vi "Line by Line Parsing Examples.vi"() -> ()   [LabVIEW 2022 SP3]
uses:
  <vilib>/regexp/Match Regular Expression.xnode
panel:
  out "Array":T1(array[cluster])
  out "before substring":string
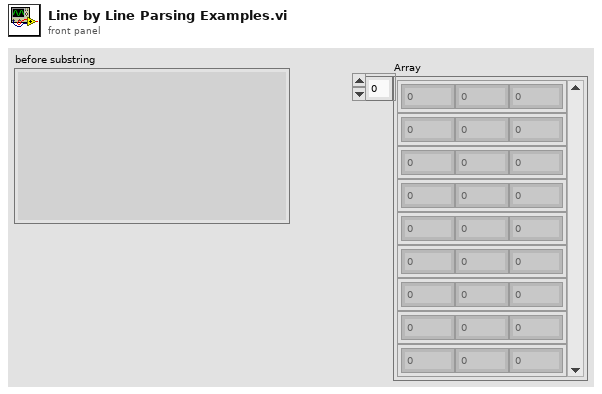
[diagram p1: front panel]
types:
  T1 = cluster{"submatch 1":i32, "submatch 2":i32, "submatch 3":i32}[]
  T2 = cluster{"submatch 1":string, "submatch 2":string, "submatch 3":string}
  T3 = cluster{"submatch 1":i32, "submatch 2":i32, "submatch 3":i32}
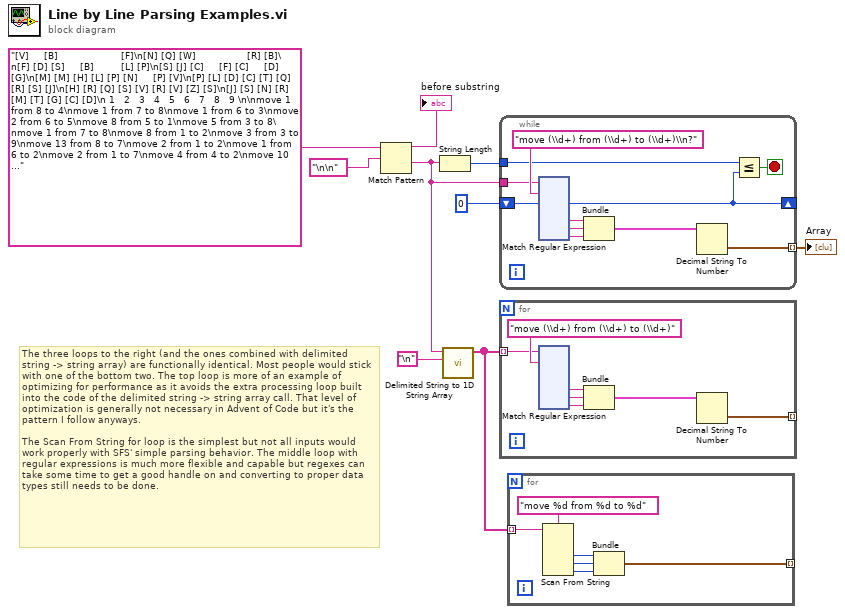
[diagram p0: block diagram]
diagram:
  # "The three loops to the right (and the ones combined with delimited string -> string array) are functionally identical. Most people would stick with one of the bottom two. The top loop is more of an example of optimizing for performance as it avoids the extra processing loop built into the code of the delimited string -> string array call. That level of optimization is generally not necessary in Advent of Code but it's the pattern I follow anyways.\n\nThe Scan From String for loop is the simplest but not all inputs would work properly with SFS' simple parsing behavior. The middle loop with regular expressions is much more flexible and capable but regexes can take some time to get a good handle on and converting to proper data types still needs to be done."
  n1 = Match Pattern(string="[V]     [B]                     [F]\n[N] [Q] [W]                 [R] [B]\n[F] [D] [S]     [B]         [L] [P]\n[S] [J] [C]     [F] [C]     [D] [G]\n[M] [M] [H] [L] [P] [N]     [P] [V]\n[P] [L] [D] [C] [T] [Q] [R] [S] [J]\n[H] [R] [Q] [S] [V] [R] [V] [Z] [S]\n[J] [S] [N] [R] [M] [T] [G] [C] [D]\n 1   2   3   4   5   6   7   8   9 \n\nmove 1 from 8 to 4\nmove 1 from 7 to 8\nmove 1 from 6 to 3\nmove 2 from 6 to 5\nmove 8 from 5 to 1\nmove 5 from 3 to 8\nmove 1 from 7 to 8\nmove 8 from 1 to 2\nmove 3 from 3 to 9\nmove 13 from 8 to 7\nmove 2 from 1 to 2\nmove 1 from 6 to 2\nmove 2 from 1 to 7\nmove 4 from 4 to 2\nmove 10 from 9 to 4\nmove 7 from 4 to 1\nmove 1 from 6 to 7\nmove 2 from 4 to 5\nmove 1 from 5 to 2\nmove 1 from 5 to 8\nmove 3 from 1 to 5\nmove 2 from 4 to 6\nmove 2 from 6 to 4\nmove 2 from 4 to 5\nmove 5 from 1 to 5\nmove 1 from 9 to 5\nmove 1 from 8 to 5\nmove 14 from 2 to 6\nmove 12 from 7 to 4\nmove 4 from 6 to 7\nmove 3 from 6 to 4\nmove 4 from 4 to 9\nmove 2 from 4 to 6\nmove 2 from 9 to 3\nmove 9 from 4 to 3\nmove 2 from 1 to 6\nmove 5 from 7 to 3\nmove 4 from 7 to 8\nmove 2 from 6 to 7\nmove 3 from 6 to 7\nmove 10 from 5 to 8\nmove 8 from 8 to 9\nmove 10 from 9 to 7\nmove 12 from 7 to 5\nmove 1 from 1 to 5\nmove 3 from 7 to 2\nmove 10 from 3 to 7\nmove 6 from 5 to 7\nmove 2 from 6 to 1\nmove 12 from 2 to 7\nmove 3 from 3 to 1\nmove 1 from 6 to 5\nmove 10 from 5 to 7\nmove 3 from 3 to 4\nmove 34 from 7 to 1\nmove 2 from 6 to 9\nmove 1 from 6 to 3\nmove 3 from 1 to 3\nmove 1 from 7 to 3\nmove 3 from 3 to 6\nmove 1 from 4 to 3\nmove 22 from 1 to 6\nmove 2 from 9 to 7\nmove 2 from 4 to 9\nmove 12 from 6 to 8\nmove 1 from 7 to 6\nmove 4 from 8 to 2\nmove 1 from 7 to 1\nmove 6 from 8 to 9\nmove 1 from 2 to 5\nmove 1 from 2 to 7\nmove 13 from 1 to 2\nmove 2 from 3 to 1\nmove 4 from 7 to 5\nmove 3 from 9 to 4\nmove 1 from 1 to 8\nmove 4 from 5 to 2\nmove 12 from 6 to 2\nmove 3 from 1 to 3\nmove 1 from 4 to 1\nmove 9 from 8 to 5\nmove 6 from 5 to 7\nmove 2 from 4 to 5\nmove 5 from 9 to 6\nmove 5 from 3 to 7\nmove 30 from 2 to 6\nmove 11 from 7 to 9\nmove 36 from 6 to 3\nmove 10 from 9 to 3\nmove 1 from 6 to 5\nmove 3 from 5 to 2\nmove 2 from 5 to 2\nmove 28 from 3 to 4\nmove 6 from 4 to 1\nmove 1 from 2 to 3\nmove 2 from 5 to 2\nmove 6 from 1 to 7\nmove 1 from 1 to 6\nmove 6 from 3 to 5\nmove 6 from 7 to 2\nmove 1 from 6 to 4\nmove 2 from 2 to 6\nmove 8 from 2 to 1\nmove 3 from 2 to 4\nmove 2 from 3 to 4\nmove 4 from 3 to 4\nmove 1 from 6 to 1\nmove 2 from 1 to 8\nmove 1 from 6 to 4\nmove 1 from 9 to 3\nmove 2 from 5 to 4\nmove 1 from 8 to 7\nmove 1 from 7 to 9\nmove 1 from 3 to 5\nmove 1 from 8 to 6\nmove 34 from 4 to 9\nmove 13 from 9 to 8\nmove 1 from 8 to 2\nmove 1 from 2 to 1\nmove 4 from 5 to 1\nmove 9 from 8 to 7\nmove 11 from 1 to 3\nmove 1 from 4 to 2\nmove 1 from 6 to 7\nmove 1 from 9 to 4\nmove 1 from 4 to 1\nmove 1 from 5 to 3\nmove 5 from 7 to 8\nmove 1 from 2 to 5\nmove 1 from 5 to 1\nmove 21 from 9 to 5\nmove 19 from 3 to 4\nmove 17 from 4 to 6\nmove 2 from 8 to 4\nmove 2 from 6 to 8\nmove 2 from 6 to 9\nmove 2 from 7 to 6\nmove 1 from 4 to 9\nmove 6 from 5 to 6\nmove 1 from 9 to 8\nmove 8 from 5 to 7\nmove 15 from 6 to 2\nmove 1 from 9 to 7\nmove 2 from 1 to 6\nmove 3 from 4 to 7\nmove 1 from 1 to 6\nmove 3 from 5 to 4\nmove 2 from 5 to 6\nmove 2 from 4 to 1\nmove 13 from 7 to 8\nmove 2 from 6 to 4\nmove 3 from 2 to 4\nmove 2 from 7 to 6\nmove 5 from 4 to 6\nmove 4 from 2 to 6\nmove 1 from 1 to 9\nmove 18 from 8 to 3\nmove 1 from 4 to 5\nmove 1 from 2 to 7\nmove 15 from 3 to 1\nmove 1 from 5 to 1\nmove 3 from 3 to 4\nmove 1 from 5 to 4\nmove 1 from 5 to 6\nmove 1 from 6 to 8\nmove 2 from 8 to 2\nmove 3 from 1 to 8\nmove 6 from 2 to 8\nmove 1 from 7 to 6\nmove 12 from 8 to 5\nmove 2 from 9 to 6\nmove 6 from 1 to 5\nmove 9 from 5 to 3\nmove 1 from 2 to 8\nmove 20 from 6 to 9\nmove 3 from 6 to 7\nmove 1 from 7 to 1\nmove 7 from 3 to 4\nmove 2 from 7 to 2\nmove 1 from 8 to 7\nmove 8 from 4 to 1\nmove 11 from 1 to 7\nmove 10 from 7 to 6\nmove 2 from 4 to 9\nmove 21 from 9 to 3\nmove 6 from 5 to 9\nmove 6 from 3 to 2\nmove 1 from 4 to 5\nmove 1 from 7 to 9\nmove 8 from 3 to 2\nmove 9 from 2 to 1\nmove 14 from 1 to 6\nmove 1 from 1 to 7\nmove 4 from 3 to 8\nmove 3 from 8 to 7\nmove 5 from 7 to 4\nmove 3 from 6 to 9\nmove 2 from 3 to 7\nmove 3 from 5 to 6\nmove 1 from 5 to 6\nmove 2 from 7 to 9\nmove 1 from 8 to 3\nmove 22 from 6 to 5\nmove 3 from 9 to 4\nmove 3 from 6 to 1\nmove 5 from 4 to 6\nmove 9 from 2 to 8\nmove 4 from 6 to 1\nmove 1 from 3 to 2\nmove 1 from 2 to 3\nmove 6 from 8 to 1\nmove 2 from 4 to 3\nmove 10 from 1 to 7\nmove 2 from 8 to 7\nmove 1 from 9 to 6\nmove 4 from 3 to 5\nmove 1 from 8 to 3\nmove 4 from 9 to 8\nmove 1 from 4 to 3\nmove 1 from 3 to 8\nmove 3 from 7 to 6\nmove 1 from 1 to 5\nmove 10 from 5 to 9\nmove 5 from 6 to 4\nmove 5 from 8 to 5\nmove 4 from 9 to 8\nmove 3 from 3 to 9\nmove 2 from 8 to 6\nmove 5 from 7 to 5\nmove 1 from 4 to 1\nmove 1 from 1 to 2\nmove 2 from 8 to 6\nmove 1 from 2 to 1\nmove 1 from 7 to 2\nmove 1 from 1 to 5\nmove 28 from 5 to 9\nmove 3 from 6 to 1\nmove 1 from 6 to 9\nmove 1 from 2 to 9\nmove 2 from 1 to 2\nmove 2 from 7 to 5\nmove 1 from 7 to 5\nmove 1 from 2 to 5\nmove 3 from 1 to 9\nmove 1 from 5 to 8\nmove 15 from 9 to 2\nmove 11 from 9 to 4\nmove 11 from 4 to 7\nmove 2 from 4 to 1\nmove 7 from 7 to 8\nmove 1 from 1 to 4\nmove 20 from 9 to 1\nmove 2 from 7 to 8\nmove 1 from 4 to 6\nmove 1 from 6 to 2\nmove 2 from 7 to 5\nmove 1 from 9 to 6\nmove 1 from 4 to 9\nmove 4 from 5 to 2\nmove 1 from 6 to 8\nmove 1 from 4 to 9\nmove 11 from 8 to 3\nmove 1 from 1 to 9\nmove 1 from 5 to 9\nmove 1 from 2 to 6\nmove 4 from 9 to 8\nmove 4 from 8 to 7\nmove 10 from 1 to 6\nmove 7 from 1 to 5\nmove 8 from 3 to 4\nmove 2 from 3 to 5\nmove 3 from 7 to 4\nmove 1 from 4 to 5\nmove 2 from 1 to 6\nmove 9 from 2 to 6\nmove 1 from 7 to 9\nmove 1 from 3 to 2\nmove 7 from 4 to 3\nmove 3 from 3 to 7\nmove 5 from 2 to 3\nmove 1 from 1 to 9\nmove 2 from 2 to 7\nmove 1 from 4 to 6\nmove 3 from 5 to 6\nmove 4 from 7 to 6\nmove 1 from 7 to 4\nmove 1 from 4 to 7\nmove 1 from 2 to 8\nmove 1 from 7 to 1\nmove 27 from 6 to 2\nmove 1 from 4 to 1\nmove 7 from 5 to 7\nmove 1 from 4 to 1\nmove 1 from 8 to 3\nmove 3 from 7 to 3\nmove 2 from 1 to 6\nmove 2 from 9 to 1\nmove 18 from 2 to 1\nmove 2 from 7 to 5\nmove 12 from 3 to 4\nmove 1 from 5 to 6\nmove 3 from 6 to 1\nmove 24 from 1 to 8\nmove 9 from 2 to 4\nmove 3 from 2 to 1\nmove 2 from 6 to 3\nmove 1 from 6 to 9\nmove 1 from 5 to 6\nmove 1 from 6 to 2\nmove 1 from 1 to 7\nmove 1 from 2 to 1\nmove 1 from 1 to 2\nmove 3 from 7 to 2\nmove 2 from 1 to 4\nmove 8 from 4 to 5\nmove 22 from 8 to 1\nmove 1 from 8 to 1\nmove 13 from 4 to 1\nmove 1 from 8 to 5\nmove 3 from 3 to 1\nmove 1 from 2 to 7\nmove 38 from 1 to 6\nmove 27 from 6 to 1\nmove 2 from 2 to 9\nmove 3 from 9 to 8\nmove 2 from 8 to 6\nmove 1 from 8 to 3\nmove 1 from 2 to 1\nmove 1 from 3 to 6\nmove 1 from 2 to 3\nmove 1 from 7 to 6\nmove 7 from 6 to 3\nmove 20 from 1 to 4\nmove 6 from 1 to 6\nmove 17 from 4 to 7\nmove 3 from 6 to 5\nmove 14 from 7 to 9\nmove 8 from 5 to 7\nmove 3 from 1 to 6\nmove 3 from 3 to 1\nmove 2 from 4 to 1\nmove 4 from 5 to 1\nmove 9 from 6 to 2\nmove 3 from 6 to 4\nmove 4 from 7 to 8\nmove 4 from 1 to 6\nmove 2 from 3 to 1\nmove 6 from 6 to 7\nmove 4 from 8 to 7\nmove 4 from 2 to 1\nmove 4 from 2 to 3\nmove 4 from 9 to 5\nmove 8 from 9 to 5\nmove 1 from 9 to 5\nmove 1 from 2 to 1\nmove 16 from 7 to 2\nmove 10 from 2 to 9\nmove 11 from 9 to 8\nmove 4 from 3 to 5\nmove 3 from 1 to 4\nmove 13 from 5 to 7\nmove 10 from 8 to 5\nmove 2 from 1 to 5\nmove 11 from 7 to 4\nmove 2 from 3 to 6\nmove 3 from 7 to 6\nmove 1 from 3 to 2\nmove 1 from 1 to 8\nmove 2 from 8 to 4\nmove 3 from 1 to 2\nmove 4 from 6 to 1\nmove 7 from 1 to 9\nmove 1 from 6 to 7\nmove 2 from 5 to 8\nmove 1 from 2 to 9\nmove 1 from 7 to 8\nmove 5 from 5 to 8\nmove 1 from 2 to 3\nmove 4 from 2 to 5\nmove 17 from 4 to 1\nmove 10 from 5 to 9\nmove 2 from 4 to 2\nmove 2 from 4 to 1\nmove 1 from 4 to 9\nmove 1 from 3 to 7\nmove 1 from 7 to 8\nmove 12 from 9 to 2\nmove 1 from 2 to 4\nmove 1 from 4 to 1\nmove 1 from 1 to 9\nmove 1 from 8 to 1\nmove 8 from 8 to 3\nmove 2 from 5 to 1\nmove 3 from 1 to 9\nmove 1 from 2 to 6\nmove 4 from 3 to 7\nmove 1 from 7 to 6\nmove 10 from 9 to 2\nmove 1 from 5 to 9\nmove 1 from 9 to 3\nmove 17 from 1 to 6\nmove 2 from 1 to 2\nmove 11 from 6 to 7\nmove 2 from 2 to 9\nmove 2 from 9 to 5\nmove 12 from 7 to 9\nmove 20 from 2 to 7\nmove 5 from 9 to 5\nmove 21 from 7 to 1\nmove 2 from 6 to 4\nmove 11 from 1 to 4\nmove 5 from 4 to 6\nmove 1 from 7 to 8\nmove 5 from 9 to 3\nmove 5 from 2 to 8\nmove 3 from 9 to 3\nmove 2 from 8 to 7\nmove 2 from 1 to 7\nmove 10 from 6 to 3\nmove 1 from 2 to 6\nmove 2 from 8 to 5\nmove 1 from 6 to 5\nmove 2 from 4 to 9\nmove 1 from 4 to 5\nmove 8 from 1 to 6\nmove 4 from 4 to 8\nmove 6 from 8 to 4\nmove 21 from 3 to 9\nmove 5 from 9 to 2\nmove 4 from 7 to 9\nmove 22 from 9 to 3\nmove 9 from 6 to 4\nmove 2 from 2 to 6\nmove 2 from 2 to 1\nmove 2 from 5 to 7\nmove 7 from 5 to 4\nmove 22 from 4 to 2\nmove 2 from 5 to 4\nmove 16 from 2 to 5\nmove 2 from 6 to 2\nmove 13 from 3 to 4\nmove 5 from 5 to 7\nmove 15 from 4 to 7\nmove 3 from 2 to 3\nmove 3 from 2 to 5\nmove 1 from 1 to 2\nmove 1 from 2 to 4\nmove 6 from 5 to 9\nmove 4 from 3 to 6\nmove 2 from 5 to 9\nmove 1 from 2 to 7\nmove 1 from 1 to 9\nmove 2 from 4 to 5\nmove 19 from 7 to 8\nmove 1 from 6 to 5\nmove 1 from 5 to 1\nmove 1 from 9 to 4\nmove 5 from 8 to 1\nmove 3 from 8 to 1\nmove 7 from 5 to 6\nmove 3 from 7 to 1\nmove 1 from 2 to 5\nmove 4 from 9 to 8\nmove 2 from 5 to 6\nmove 10 from 1 to 4\nmove 1 from 7 to 2\nmove 6 from 3 to 4\nmove 9 from 4 to 3\nmove 2 from 2 to 8\nmove 2 from 9 to 5\nmove 5 from 8 to 3\nmove 1 from 1 to 5\nmove 2 from 5 to 6\nmove 1 from 1 to 7\nmove 2 from 9 to 7\nmove 8 from 4 to 7\nmove 3 from 3 to 9\nmove 4 from 6 to 3\nmove 1 from 5 to 3\nmove 1 from 7 to 2\nmove 1 from 2 to 1\nmove 1 from 6 to 5\nmove 1 from 5 to 2\nmove 10 from 7 to 4\nmove 10 from 4 to 1\nmove 10 from 1 to 8\nmove 1 from 9 to 6\nmove 1 from 1 to 4\nmove 11 from 8 to 1\nmove 2 from 9 to 5\nmove 5 from 6 to 3\nmove 1 from 3 to 8\nmove 4 from 1 to 3\nmove 5 from 3 to 8\nmove 1 from 4 to 7\nmove 1 from 7 to 2\nmove 13 from 3 to 5\nmove 2 from 2 to 1\nmove 4 from 3 to 1\nmove 4 from 5 to 6\nmove 3 from 6 to 2\nmove 4 from 5 to 4\nmove 8 from 8 to 7\nmove 1 from 3 to 9", regular expression="\n\n") -> (before substring=→"before substring":string, after substring=w3:string)  [unwired: 1 in, 2 out]
  n2 = String Length(string=w3) -> (length=w4:i32)
  n3 = call <vilib>:"Delimited String to 1D String Array.vi"("delimiter"="\n", "delimited string"=w3) -> ("string array"=w1:string[])  [unwired: 9 in]
  n4 = while {
    tunnel: [w15] -> w6 mode=indexing
    tunnel: w3 -> [w14]
    shift-right: [w11] -> _
    shift-left: 0 -> [w13]
    tunnel: w4 -> [w12]
    stop <- w10 stop-if-true
    n5 = xnode "Match Regular Expression"("input string"=w14, "regular expression"="move (\\d+) from (\\d+) to (\\d+)\\n?", "offset (0)"=w13) -> ("offset past match"=w11:i32, "submatch 1"=w19:string, "submatch 2"=w18:string, "submatch 3"=w17:string)  [unwired: 3 in, 4 out]
    n6 = Bundle("submatch 1"=w19, "submatch 2"=w18, "submatch 3"=w17) -> (w16:T2)  [unwired: 1 in]
    n7 = Decimal String To Number(string=w16) -> (number=w15:T3)  [unwired: 2 in, 1 out]
    n8 = Less Or Equal?(x=w12, y=w11) -> (x <= y?=w10:bool)
  }
  "Array" <- w6
  n9 = for {
    tunnel: [w143] -> _ mode=indexing
    tunnel: w1 -> [w142] mode=indexing
    n10 = xnode "Match Regular Expression"("input string"=w142, "regular expression"="move (\\d+) from (\\d+) to (\\d+)") -> ("submatch 1"=w147:string, "submatch 2"=w146:string, "submatch 3"=w145:string)  [unwired: 4 in, 5 out]
    n11 = Bundle("submatch 1"=w147, "submatch 2"=w146, "submatch 3"=w145) -> (w144:T2)  [unwired: 1 in]
    n12 = Decimal String To Number(string=w144) -> (number=w143:T3)  [unwired: 2 in, 1 out]
  }
  n13 = for {
    tunnel: w1 -> [w275] mode=indexing
    tunnel: [w270] -> _ mode=indexing
    n14 = Scan From String(format string="move %d from %d to %d", input string=w275) -> (output 1=w273:i32, output 2=w272:i32, output 3=w271:i32)  [unwired: 5 in, 3 out]
    n15 = Bundle(w273, w272, w271) -> (w270:cluster{i32, i32, i32})  [unwired: 1 in]
  }
